vi "SensorDAQ.vi"   [LabVIEW 2017]
panel:
  # "This is responsible for aquiering data from all sensors"
  # "Each sensor should publish data to a queue via a \"lossy enqueue element\" vi\nand be set with a max queue size."
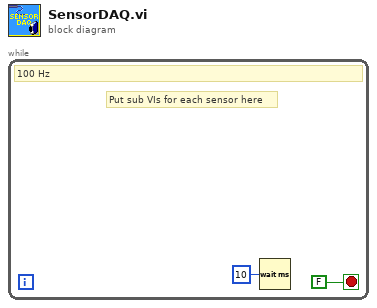
[diagram p0: block diagram]
diagram:
  n1 = while {
    stop <- FALSE stop-if-true
    # "Put sub VIs for each sensor here"
    # "100 Hz"
    n2 = Wait (ms)(milliseconds to wait=u32 10) -> ()  [unwired: 1 out]
  }
